vi "configurations to from repo cluster.vi"(8 "error in":errorcluster, 11 "configurations":refnum<class "NISE_CEF_serializable configuration.lvclass">[](array[class])) -> (0 "error out":errorcluster, 3 "from repo cluster":T1)   [LabVIEW 2013, in "NISE_CEF_serializable node.lvclass"]
uses:
  NISE_CEF_serializable node.lvclass
  Node/FromRepoCluster.ctl
  serializable configuration/NISE_CEF_serializable configuration.lvclass
  Node/NISE_CEF_Node.lvclass
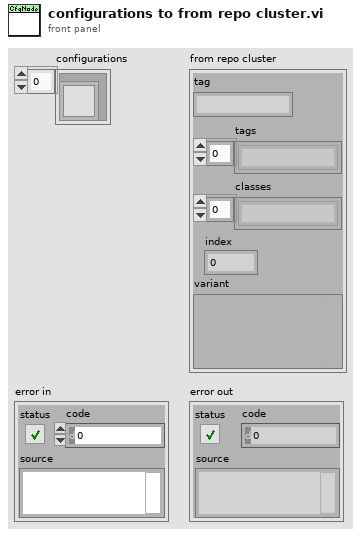
[diagram p1: front panel]
types:
  T1 = typedef "NISE_CEF_Node.lvclass/FromRepoCluster.ctl" = cluster{"tag":string, "tags":string[], "classes":string[], "index":i32, "variant":variant}
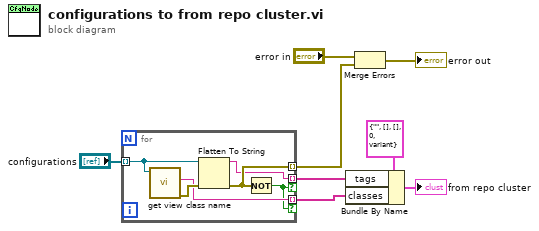
[diagram p0: block diagram]
diagram:
  n1 = for {
    tunnel: "configurations" -> [w14] mode=indexing
    tunnel: [w12] -> w6 mode=indexing
    tunnel: [w11] -> w1 mode=indexing if=w9
    tunnel: [w10] -> w2 mode=indexing if=w9
    n2 = call "get view class name.vi"("configuration in"=w14) -> ("error out"=w13:errorcluster, "view class"=w11:string)  [unwired: 8 in, 1 out]
    n3 = Flatten To String(anything=w14, error in (no error)=w13) -> (data string=w10:string, error out=w12:errorcluster)  [unwired: 2 in, 1 out]
    n4 = Not(x=w12) -> (.not. x?=w9:bool)
  }
  n5 = Bundle By Name(cluster=T1 {"tag"="", "tags"=[], "classes"=[], "index"=0, "variant"=variant} ("from repo cluster"), "tags"=w2, "classes"=w1) -> (→"from repo cluster":T1)
  n6 = Merge Errors("error in", w6) -> (→"error out":errorcluster)
